vi "EnableDiasableIncrement.vi"(8 "Increment Buttons":refnum<vi>, 10 "Increment":string, 11 "Position":cluster{"Card":dbl, "Channel":dbl}) -> ()   [LabVIEW 2013]
doc: "Increments or Decrements Delay Time when + or - is clicked.\nSets + and - buttons to 'enabled' (clickable) when 'Manual' is selected\n\n-Programmer Note:\nIn case this doesn't work, look at comparing old value with new value for update"
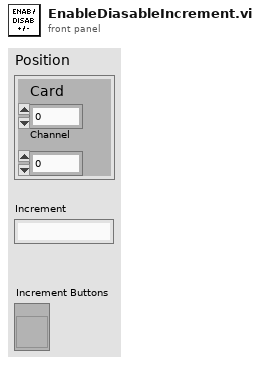
[diagram p1: front panel]
types:
  T1 = enum8{"Enabled", "Disabled", "Disabled and Grayed Out"}
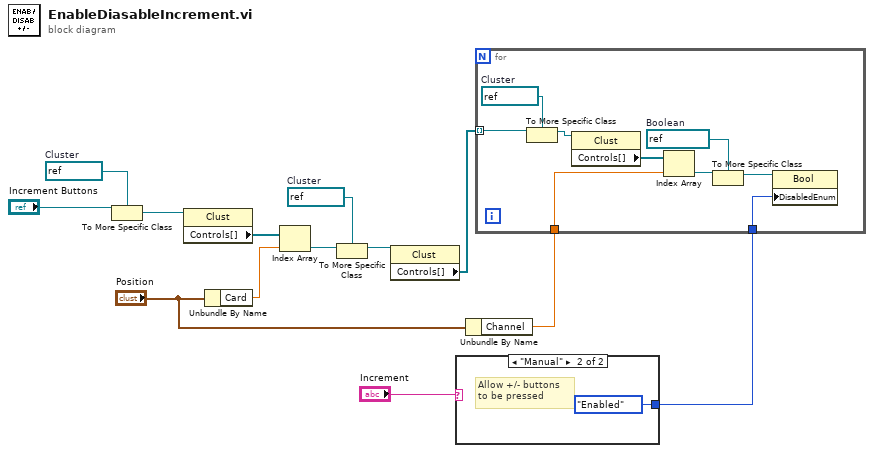
[diagram p0: block diagram]
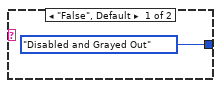
[diagram p2: hidden frame]
diagram:
  w6 = refnum<vi> refnum  # Cluster
  w11 = refnum<vi> refnum  # Cluster
  n1 = To More Specific Class(target class=w11, reference="Increment Buttons") -> (specific class reference=w10:refnum<vi>)  [unwired: 1 in, 1 out]
  n2 = property class="Clust"(reference=w10) -> ("Controls[]"=w9:refnum<vi>[])  [unwired: 1 in, 2 out]
  n3 = Unbundle By Name("Position") -> ("Card"=w8:dbl)
  n4 = Index Array(array=w9, index=w8) -> (element=w7:refnum<vi>)
  n5 = To More Specific Class(target class=w6, reference=w7) -> (specific class reference=w5:refnum<vi>)  [unwired: 1 in, 1 out]
  n6 = property class="Clust"(reference=w5) -> ("Controls[]"=w4:refnum<vi>[])  [unwired: 1 in, 2 out]
  n7 = case shown="\"Manual\"" "Increment" {
    tunnel: [T1."Disabled and Grayed Out" ("Disabled") T1."Enabled" ("Disabled")] -> w1
    frame "False", Default {
    }
    frame "Manual" {
      # "Allow +/- buttons\nto be pressed"
    }
  }
  n8 = Unbundle By Name("Position") -> ("Channel"=w2:dbl)
  n9 = for {
    tunnel: w4 -> [w24] mode=indexing
    tunnel: w2 -> [w20]
    tunnel: w1 -> [w16]
    w18 = refnum<vi> refnum  # Boolean
    w23 = refnum<vi> refnum  # Cluster
    n10 = To More Specific Class(target class=w23, reference=w24) -> (specific class reference=w22:refnum<vi>)  [unwired: 1 in, 1 out]
    n11 = property class="Clust"(reference=w22) -> ("Controls[]"=w21:refnum<vi>[])  [unwired: 1 in, 2 out]
    n12 = Index Array(array=w21, index=w20) -> (element=w19:refnum<vi>)
    n13 = To More Specific Class(target class=w18, reference=w19) -> (specific class reference=w17:refnum<vi>)  [unwired: 1 in, 1 out]
    n14 = property class="Bool"(reference=w17, "DisabledEnum"=w16) -> ()  [unwired: 1 in, 2 out]
  }
